vi "Channel ID to Tree Items.vi"(8 "error in (no error)":errorcluster, 9 "Channel ID":string, 11 "Application Data in":T2) -> (0 "error out":errorcluster, 1 "Settings":T1, 2 "Item":T1, 3 "Application Data out":T2)   [LabVIEW 2017, in "DSF Configuration Utility.lvlib"]
uses:
  DSF Configuration Utility.lvlib
  Main VI/Application Data.ctl
  <vilib>/National Instruments/Data Sharing Framework Core/Data Sharing Framework Core.lvlibp/Configuration/1.0.0/Public/Controls/DSF Config Data RefNum.ctl
  Main VI/View Mode.ctl
  Tree Item.ctl
  Tree Item Type.ctl
  <vilib>/National Instruments/Data Sharing Framework Core/Data Sharing Framework Core.lvlibp/Configuration/1.0.0/Public/Read Item/Read Settings.vi
  <vilib>/National Instruments/Data Sharing Framework Core/Data Sharing Framework Core.lvlibp/Configuration/1.0.0/Public/Read Item/Read Channel.vi
  <vilib>/National Instruments/Data Sharing Framework Core/Data Sharing Framework Core.lvlibp/Configuration/1.0.0/Data Sharing Framework Configuration.lvlib
panel:
  # "App\nData"
  # "App\nData"
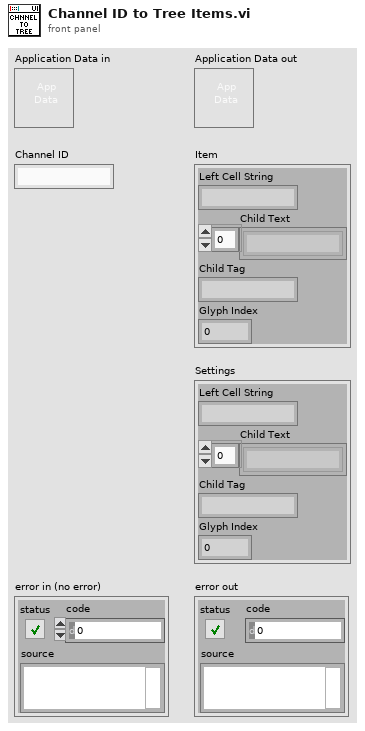
[diagram p1: front panel]
types:
  T1 = typedef "DSF Configuration Utility.lvlib/Tree Item.ctl" = cluster{"Left Cell String":string, "Child Text":string[], "Child Tag":string, "Glyph Index":i32}
  T2 = typedef "DSF Configuration Utility.lvlib/Application Data.ctl" = cluster{"Item Tree Control":refnum<vi>, "Value Tree Control":refnum<vi>, "DSF Refnum":T3, "Top-Level VI":refnum<vi>, "View State":T4, "menu reference":refnum<k9>}
  T3 = typedef "Data Sharing Framework Core.lvlibp/Data Sharing Framework Configuration.lvlib/DSF Config Data RefNum.ctl" = refnum<k1>
  T4 = typedef "DSF Configuration Utility.lvlib/View Mode.ctl" = enum16{"Tree", "List"}
  T5 = typedef "DSF Configuration Utility.lvlib/Tree Item Type.ctl" = enum16{"Plugin", "Group", "Transfer", "Channel", "Setting"}
  T6 = typedef "Data Sharing Framework Core.lvlibp/Data Sharing Framework Configuration.lvlib/DSF Channel Info.ctl" = cluster{"count":u64, "buffer offset":u64, "data type":T7, "settings id":string}
  T7 = typedef "Data Sharing Framework Core.lvlibp/Data Sharing Framework Configuration.lvlib/DSF Data Type.ctl" = enum8{"Bool", "SGL", "DBL", "I8", "I16", "I32", "I64", "U8", "U16", "U32", "U64"}
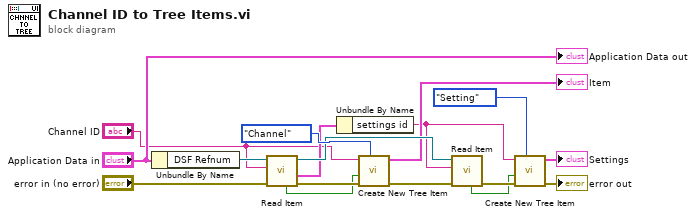
[diagram p0: block diagram]
diagram:
  n1 = Unbundle By Name("Application Data in") -> ("DSF Refnum"=w8:T3)
  n2 = call-poly <vilib>:"Read Item.vi"("error in (no error)"="error in (no error)", "Channel ID"="Channel ID", "dsf refnum"=w8) -> ("error out"=w12:errorcluster, "value"=w9:T6, "dsf refnum out"=w10:T3, "found?"=w3:bool)  [unwired: 5 in]
  n3 = Unbundle By Name(w9) -> ("settings id"=w2:string)
  n4 = call "Create New Tree Item.vi"("Item Type"=Tree_Item_Type."Channel", "error in"=w12, "found?"=w3, "Left Cell String"="Channel ID") -> ("error out"=w13:errorcluster, "Item"=→"Item":T1)  [unwired: 6 in]
  n5 = call-poly <vilib>:"Read Item.vi"("error in (no error)"=w13, "Settings ID"=w2, "dsf refnum"=w10) -> ("error out"=w14:errorcluster, "found?"=w1:bool)  [unwired: 5 in, 2 out]
  n6 = call "Create New Tree Item.vi"("Item Type"=Tree_Item_Type."Setting", "error in"=w14, "found?"=w1, "Left Cell String"=w2) -> ("error out"=→"error out":errorcluster, "Item"=→"Settings":T1)  [unwired: 6 in]
  "Application Data out" <- "Application Data in"
